vi "UI_Design.vi"() -> ()   [LabVIEW 2023]
uses:
  Vertical_Point_Slide.ctl
  Vertical_Flat_Slide.ctl
  Boolean.ctl
  Numeric.ctl
  String.ctl
  Combo_Box.ctl
  List_Box.ctl
  Ok_Boolean.ctl
  Gauge.ctl
  Waveform_Graph.ctl
  <vilib>/Analysis/NI_AALBase.lvlib
panel:
  out "Waveform_Chart":T1=[0.0, 0.049067674327418015, 0.0980171403295606, 0.14673047445536175, 0.19509032201612828, 0.2429801799032639, 0.2902846772544624, 0.33688985339222005, 0.38268343236508984, 0.4275550934302821, 0.4713967368259977, 0.5141027441932218, 0.5555702330196023, 0.5956993044924334, 0.6343932841636456, 0.6715589548470184, 0.7071067811865477, 0.7409511253549591, 0.7730104533627371, 0.8032075314806449, 0.8314696123025453, 0.8577286100002721, 0.8819212643483552, 0.9039892931234434, 0.923879532511287, 0.9415440651830209, 0.956940335732209, 0.9700312531945442, 0.9807852804032307, 0.9891765099647812, 0.9951847266721972, 0.9987954562051726, 1.0, 0.9987954562051726, 0.9951847266721969, 0.9891765099647812, 0.9807852804032305, 0.9700312531945443, 0.9569403357322089, 0.9415440651830211, 0.9238795325112868, 0.9039892931234437, 0.8819212643483552, 0.8577286100002723, 0.8314696123025453, 0.8032075314806452, 0.7730104533627371, 0.7409511253549593, 0.7071067811865477, 0.6715589548470187, 0.6343932841636457, 0.5956993044924336, 0.5555702330196024, 0.5141027441932219, 0.4713967368259978, 0.4275550934302822, 0.38268343236508995, 0.3368898533922201, 0.29028467725446255, 0.24298017990326393, 0.19509032201612847, 0.14673047445536175, 0.0980171403295608, 0.04906767432741799, 1.942890293094024e-16, -0.04906767432741807, -0.09801714032956041, -0.14673047445536183, -0.19509032201612808, -0.24298017990326398, -0.29028467725446216, -0.33688985339222016, -0.3826834323650896, -0.4275550934302822, -0.4713967368259975, -0.5141027441932219, -0.5555702330196021, -0.5956993044924335, -0.6343932841636454, -0.6715589548470186, -0.7071067811865475, -0.7409511253549592, -0.7730104533627369, -0.803207531480645, -0.8314696123025451, -0.8577286100002722, -0.8819212643483549, -0.9039892931234434, -0.9238795325112867, -0.9415440651830209, -0.9569403357322088, -0.9700312531945442, -0.9807852804032304, -0.9891765099647812, -0.9951847266721969, -0.9987954562051726, -1.0, -0.9987954562051726, -0.9951847266721969, -0.9891765099647812, -0.9807852804032305, -0.9700312531945443, -0.9569403357322089, -0.9415440651830211, -0.9238795325112868, -0.9039892931234437, -0.8819212643483552, -0.8577286100002723, -0.8314696123025453, -0.8032075314806452, -0.7730104533627371, -0.7409511253549593, -0.7071067811865477, -0.6715589548470187, -0.6343932841636457, -0.5956993044924336, -0.5555702330196024, -0.5141027441932219, -0.4713967368259978, -0.4275550934302822, -0.38268343236508995, -0.3368898533922201, -0.29028467725446255, -0.24298017990326393, -0.19509032201612847, -0.14673047445536175, -0.0980171403295608, -0.04906767432741799]
  out "Gauge":T2 scale=0.0..10.0
  in  "OK_Button":T3
  in  "Boolean_2":T4
  in  "Listbox":T5
  in  "Combo Box":T6
  out "String":T7
  in  "Numeric":T8
  in  "Path":path
  in  "Boolean":T4
  in  "Vertical_Flat_Slide":T9 scale=0.0..10.0
  in  "Vertical_Point_Slide":T10 scale=0.0..10.0
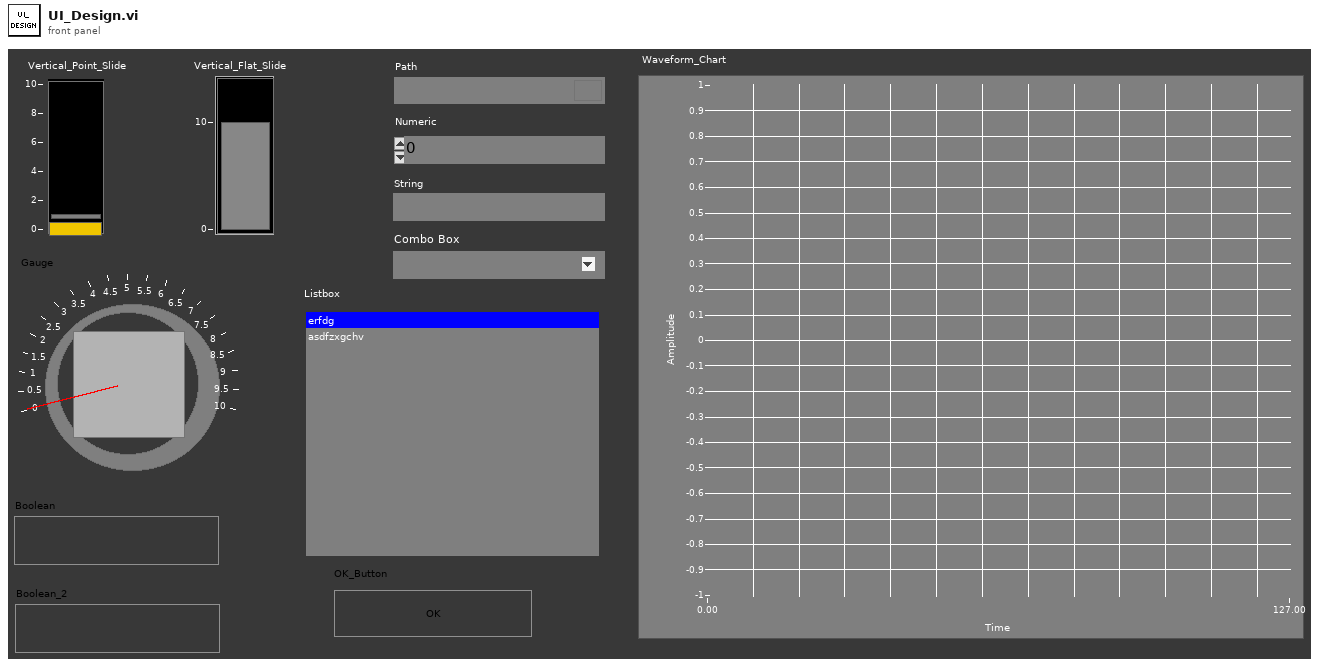
[diagram p1: front panel]
types:
  T1 = typedef "Waveform_Graph.ctl" = dbl[]
  T2 = typedef "Gauge.ctl" = dbl
  T3 = typedef "Ok_Boolean.ctl" = bool
  T4 = typedef "Boolean.ctl" = bool
  T5 = typedef "List_Box.ctl" = i32
  T6 = typedef "Combo_Box.ctl" = string
  T7 = typedef "String.ctl" = string
  T8 = typedef "Numeric.ctl" = dbl
  T9 = typedef "Vertical_Flat_Slide.ctl" = dbl
  T10 = typedef "Vertical_Point_Slide.ctl" = dbl
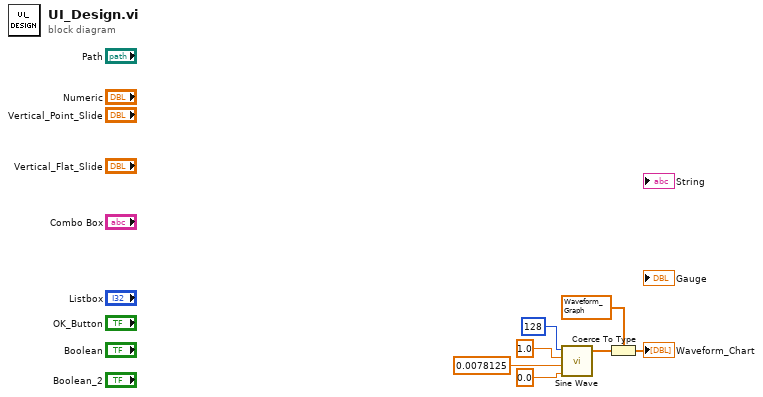
[diagram p0: block diagram]
diagram:
  n1 = call <vilib>:"Sine Wave.vi"("samples"=128, "amplitude"=1.0, "frequency"=0.0078125, "phase in"=0.0) -> ("sine wave"=w3:dbl[])  [unwired: 1 in, 2 out]
  n2 = Coerce To Type(0:w3, 1:T1 [0.0, 0.049067674327418015, 0.0980171403295606, 0.14673047445536175, 0.19509032201612828, 0.2429801799032639, 0.2902846772544624, 0.33688985339222005, 0.38268343236508984, 0.4275550934302821, 0.4713967368259977, 0.5141027441932218, 0.5555702330196023, 0.5956993044924334, 0.6343932841636456, 0.6715589548470184, 0.7071067811865477, 0.7409511253549591, 0.7730104533627371, 0.8032075314806449, 0.8314696123025453, 0.8577286100002721, 0.8819212643483552, 0.9039892931234434, 0.923879532511287, 0.9415440651830209, 0.956940335732209, 0.9700312531945442, 0.9807852804032307, 0.9891765099647812, 0.9951847266721972, 0.9987954562051726, 1.0, 0.9987954562051726, 0.9951847266721969, 0.9891765099647812, 0.9807852804032305, 0.9700312531945443, 0.9569403357322089, 0.9415440651830211, 0.9238795325112868, 0.9039892931234437, 0.8819212643483552, 0.8577286100002723, 0.8314696123025453, 0.8032075314806452, 0.7730104533627371, 0.7409511253549593, 0.7071067811865477, 0.6715589548470187, 0.6343932841636457, 0.5956993044924336, 0.5555702330196024, 0.5141027441932219, 0.4713967368259978, 0.4275550934302822, 0.38268343236508995, 0.3368898533922201, 0.29028467725446255, 0.24298017990326393, 0.19509032201612847, 0.14673047445536175, 0.0980171403295608, 0.04906767432741799, 1.942890293094024e-16, -0.04906767432741807, -0.09801714032956041, -0.14673047445536183, -0.19509032201612808, -0.24298017990326398, -0.29028467725446216, -0.33688985339222016, -0.3826834323650896, -0.4275550934302822, -0.4713967368259975, -0.5141027441932219, -0.5555702330196021, -0.5956993044924335, -0.6343932841636454, -0.6715589548470186, -0.7071067811865475, -0.7409511253549592, -0.7730104533627369, -0.803207531480645, -0.8314696123025451, -0.8577286100002722, -0.8819212643483549, -0.9039892931234434, -0.9238795325112867, -0.9415440651830209, -0.9569403357322088, -0.9700312531945442, -0.9807852804032304, -0.9891765099647812, -0.9951847266721969, -0.9987954562051726, -1.0, -0.9987954562051726, -0.9951847266721969, -0.9891765099647812, -0.9807852804032305, -0.9700312531945443, -0.9569403357322089, -0.9415440651830211, -0.9238795325112868, -0.9039892931234437, -0.8819212643483552, -0.8577286100002723, -0.8314696123025453, -0.8032075314806452, -0.7730104533627371, -0.7409511253549593, -0.7071067811865477, -0.6715589548470187, -0.6343932841636457, -0.5956993044924336, -0.5555702330196024, -0.5141027441932219, -0.4713967368259978, -0.4275550934302822, -0.38268343236508995, -0.3368898533922201, -0.29028467725446255, -0.24298017990326393, -0.19509032201612847, -0.14673047445536175, -0.0980171403295608, -0.04906767432741799] ("Waveform_Chart")) -> (2:→"Waveform_Chart":T1)
